vi "LaserMonitorLDC501.vi"() -> ()   [LabVIEW 2020]
panel:
  in  "Internal Trigger Rate (1 MHz)":i32=1000000 min=0 max=10000000
  out "VISA resource name out":refnum<visa-resource-name>
  out "error out":errorcluster
  in  "error in (no error)":errorcluster
  in  "VISA resource name":refnum<visa-resource-name>
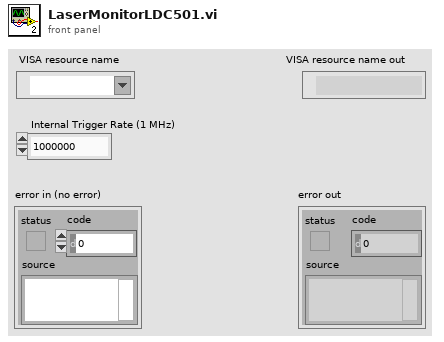
[diagram p1: front panel]
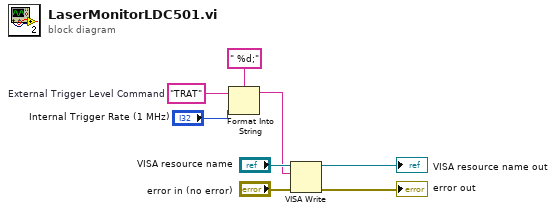
[diagram p0: block diagram]
diagram:
  w6 = "TRAT"  # External Trigger Level Command
  n1 = Format Into String(format string=" %d;" ("Source Command"), initial string=w6, "Internal Trigger Rate (1 MHz)") -> (resulting string=w3:string)  [unwired: 1 in, 1 out]
  n2 = VISA Write(VISA resource name="VISA resource name", write buffer=w3, error in (no error)="error in (no error)") -> (VISA resource name out=→"VISA resource name out":refnum<visa-resource-name>, error out=→"error out":errorcluster)  [unwired: 1 out]
